vi "InitConfig.vi"   [LabVIEW 2011]
uses:
  <vilib>/Utility/config.llb/Write Key (Double).vi
  <vilib>/Utility/config.llb/Write Key (I32).vi
  <vilib>/Utility/config.llb/Write Key (String).vi
  <vilib>/Utility/config.llb/NI_LVConfig.lvlib
types:
  T1 = typedef "NI_LVConfig.lvlib/Config Data RefNum.ctl" = refnum<k1>
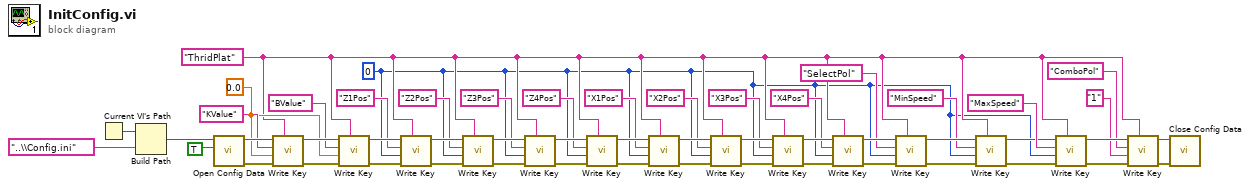
[diagram p0: block diagram]
diagram:
  w2 = 0
  w6 = "ThridPlat" ("section")
  w18 = 0.0
  n1 = Current VI's Path() -> (path=w52:path)
  n2 = Build Path(base path=w52, name or relative path="..\\Config.ini" ("名称或相对路径")) -> (appended path=w50:path)
  n3 = call <vilib>:"Open Config Data.vi"("create file if necessary (T)"=TRUE, "configuration file path"=w50) -> ("error out"=w46:errorcluster, "refnum"=w48:T1)  [unwired: 7 in, 1 out]
  n4 = call-poly <vilib>:"Write Key.vi"("section"=w6, "error in (no error)"=w46, "value"=w18, "key"="KValue", "refnum"=w48) -> ("error out"=w44:errorcluster, "refnum out"=w45:T1)  [unwired: 4 in, 1 out]
  n5 = call-poly <vilib>:"Write Key.vi"("section"=w6, "error in (no error)"=w44, "value"=w18, "key"="BValue", "refnum"=w45) -> ("error out"=w42:errorcluster, "refnum out"=w41:T1)  [unwired: 4 in, 1 out]
  n6 = call-poly <vilib>:"Write Key.vi"("section"=w6, "error in (no error)"=w42, "value"=w2, "key"="Z1Pos", "refnum"=w41) -> ("error out"=w39:errorcluster, "refnum out"=w38:T1)  [unwired: 4 in, 1 out]
  n7 = call-poly <vilib>:"Write Key.vi"("section"=w6, "error in (no error)"=w39, "value"=w2, "key"="Z2Pos", "refnum"=w38) -> ("error out"=w36:errorcluster, "refnum out"=w37:T1)  [unwired: 4 in, 1 out]
  n8 = call-poly <vilib>:"Write Key.vi"("section"=w6, "error in (no error)"=w36, "value"=w2, "key"="Z3Pos", "refnum"=w37) -> ("error out"=w34:errorcluster, "refnum out"=w35:T1)  [unwired: 4 in, 1 out]
  n9 = call-poly <vilib>:"Write Key.vi"("section"=w6, "error in (no error)"=w34, "value"=w2, "key"="Z4Pos", "refnum"=w35) -> ("error out"=w32:errorcluster, "refnum out"=w33:T1)  [unwired: 4 in, 1 out]
  n10 = call-poly <vilib>:"Write Key.vi"("section"=w6, "error in (no error)"=w32, "value"=w2, "key"="X1Pos", "refnum"=w33) -> ("error out"=w30:errorcluster, "refnum out"=w31:T1)  [unwired: 4 in, 1 out]
  n11 = call-poly <vilib>:"Write Key.vi"("section"=w6, "error in (no error)"=w30, "value"=w2, "key"="X2Pos", "refnum"=w31) -> ("error out"=w28:errorcluster, "refnum out"=w29:T1)  [unwired: 4 in, 1 out]
  n12 = call-poly <vilib>:"Write Key.vi"("section"=w6, "error in (no error)"=w28, "value"=w2, "key"="X3Pos", "refnum"=w29) -> ("error out"=w26:errorcluster, "refnum out"=w27:T1)  [unwired: 4 in, 1 out]
  n13 = call-poly <vilib>:"Write Key.vi"("section"=w6, "error in (no error)"=w26, "value"=w2, "key"="X4Pos", "refnum"=w27) -> ("error out"=w16:errorcluster, "refnum out"=w17:T1)  [unwired: 4 in, 1 out]
  n14 = call-poly <vilib>:"Write Key.vi"("section"=w6, "error in (no error)"=w16, "value"=w2, "key"="SelectPol", "refnum"=w17) -> ("error out"=w14:errorcluster, "refnum out"=w15:T1)  [unwired: 4 in, 1 out]
  n15 = call-poly <vilib>:"Write Key.vi"("section"=w6, "error in (no error)"=w14, "value"=w2, "key"="MinSpeed", "refnum"=w15) -> ("error out"=w9:errorcluster, "refnum out"=w10:T1)  [unwired: 4 in, 1 out]
  n16 = call-poly <vilib>:"Write Key.vi"("section"=w6, "error in (no error)"=w9, "value"=w2, "key"="MaxSpeed", "refnum"=w10) -> ("error out"=w7:errorcluster, "refnum out"=w8:T1)  [unwired: 4 in, 1 out]
  n17 = call-poly <vilib>:"Write Key.vi"("section"=w6, "error in (no error)"=w7, "value"="1", "key"="ComboPol", "refnum"=w8) -> ("error out"=w3:errorcluster, "refnum out"=w4:T1)  [unwired: 4 in, 1 out]
  n18 = call <vilib>:"Close Config Data.vi"("error in (no error)"=w3, "refnum"=w4) -> ()  [unwired: 1 in, 9 out]
